vi "Calculate Error.vi"(8 "Rear Right":T1, 9 "Rear Left":T1, 10 "Front Left":T1, 11 "Front Right":T1) -> (0 "Rear Right Angle Error":dbl, 1 "Rear Left Angle Error":dbl, 2 "Rear Right Drive Power":dbl, 3 "Rear Left Drive Power":dbl, 4 "Front Left Angle Error":dbl, 5 "Front Left Drive Power":dbl, 6 "Front Right Angle Error":dbl, 7 "Front Right Drive Power":dbl)   [LabVIEW 2018]
uses:
  Final Motor Data.ctl
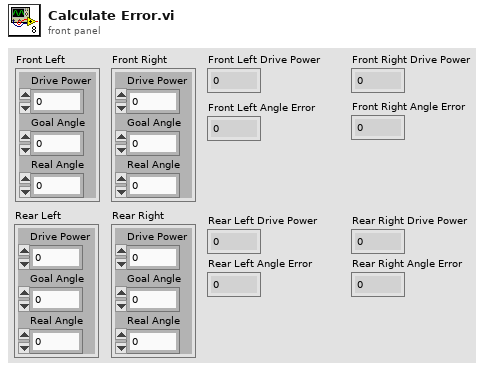
[diagram p1: front panel]
types:
  T1 = typedef "Final Motor Data.ctl" = cluster{"Drive Power":dbl, "Goal Angle":dbl, "Real Angle":dbl}
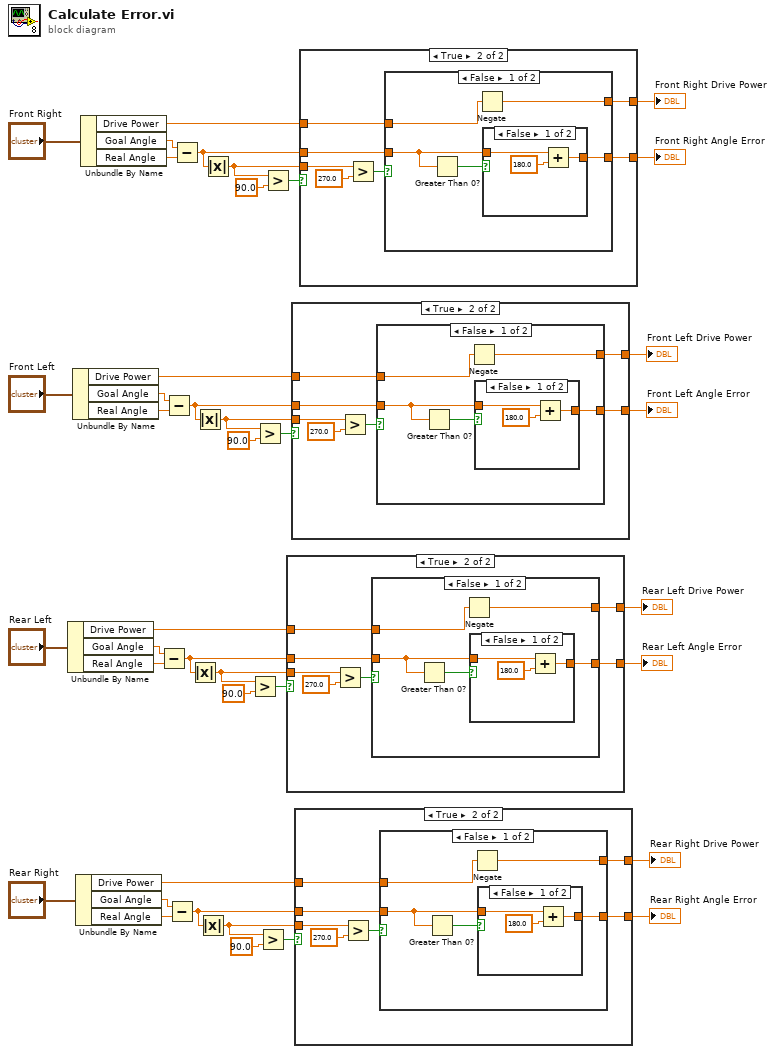
[diagram p0: block diagram]
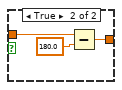
[diagram p3: hidden frame]
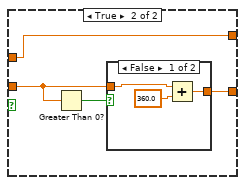
[diagram p4: hidden frame]
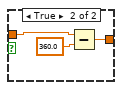
[diagram p5: hidden frame]
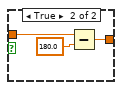
[diagram p7: hidden frame]
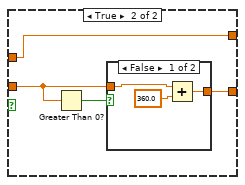
[diagram p8: hidden frame]
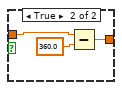
[diagram p9: hidden frame]
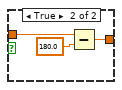
[diagram p11: hidden frame]
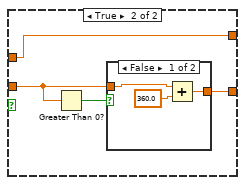
[diagram p12: hidden frame]
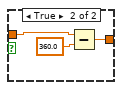
[diagram p13: hidden frame]
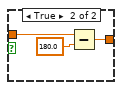
[diagram p15: hidden frame]
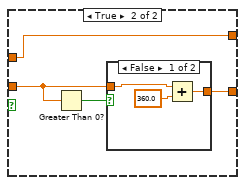
[diagram p16: hidden frame]
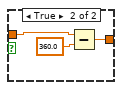
[diagram p17: hidden frame]
diagram:
  n1 = Unbundle By Name("Rear Left") -> ("Drive Power"=w6:dbl, "Goal Angle"=w5:dbl, "Real Angle"=w4:dbl)
  n2 = Unbundle By Name("Front Left") -> ("Drive Power"=w9:dbl, "Goal Angle"=w8:dbl, "Real Angle"=w7:dbl)
  n3 = Unbundle By Name("Rear Right") -> ("Drive Power"=w3:dbl, "Goal Angle"=w2:dbl, "Real Angle"=w1:dbl)
  n4 = Unbundle By Name("Front Right") -> ("Drive Power"=w10:dbl, "Goal Angle"=w12:dbl, "Real Angle"=w11:dbl)
  n5 = Subtract(x=w5, y=w4) -> (x-y=w21:dbl)
  n6 = Subtract(x=w8, y=w7) -> (x-y=w27:dbl)
  n7 = Subtract(x=w2, y=w1) -> (x-y=w15:dbl)
  n8 = Subtract(x=w12, y=w11) -> (x-y=w33:dbl)
  n9 = Absolute Value(x=w21) -> (abs(x)=w22:dbl)
  n10 = Absolute Value(x=w27) -> (abs(x)=w28:dbl)
  n11 = Absolute Value(x=w15) -> (abs(x)=w16:dbl)
  n12 = Absolute Value(x=w33) -> (abs(x)=w34:dbl)
  n13 = Greater?(x=w22, y=90.0) -> (0:w23:bool)
  n14 = Greater?(x=w28, y=90.0) -> (0:w29:bool)
  n15 = Greater?(x=w16, y=90.0) -> (0:w17:bool)
  n16 = Greater?(x=w34, y=90.0) -> (0:w35:bool)
  n17 = case shown="True" w23 {
    tunnel: w22 -> [_ w49]
    tunnel: w6 -> [w42 w46]
    tunnel: [w42 w43] -> w20
    tunnel: [w41 w44] -> w19
    tunnel: w21 -> [w41 w45]
    frame False {
      # "Choice D: NO CHANGE"
    }
    frame True {
      n18 = Greater?(x=w49, y=270.0) -> (0:w47:bool)
      n19 = case shown="False" w47 {
        tunnel: w46 -> [w54 w61]
        tunnel: w45 -> [w51 w63]
        tunnel: [w50 w62] -> w44
        tunnel: [w53 w61] -> w43
        frame False {
          n20 = Greater Than 0?(x=w51) -> (x > 0?=w52:bool)
          n21 = Negate(x=w54) -> (-x=w53:dbl)
          n22 = case shown="False" w52 {
            tunnel: w51 -> [w56 w59]
            tunnel: [w55 w58] -> w50
            frame False {
              n23 = Add(x=w56, y=180.0) -> (x+y=w55:dbl)
            }
            frame True {
              n24 = Subtract(x=w59, y=180.0) -> (x-y=w58:dbl)
            }
          }
        }
        frame True {
          n25 = Greater Than 0?(x=w63) -> (x > 0?=w64:bool)
          n26 = case shown="False" w64 {
            tunnel: w63 -> [w66 w69]
            tunnel: [w65 w68] -> w62
            frame False {
              n27 = Add(x=w66, y=360.0) -> (x+y=w65:dbl)
            }
            frame True {
              n28 = Subtract(x=w69, y=360.0) -> (x-y=w68:dbl)
            }
          }
        }
      }
    }
  }
  "Rear Left Drive Power" <- w20
  "Rear Left Angle Error" <- w19
  n29 = case shown="True" w29 {
    tunnel: w28 -> [_ w79]
    tunnel: w9 -> [w72 w76]
    tunnel: [w72 w73] -> w26
    tunnel: [w71 w74] -> w25
    tunnel: w27 -> [w71 w75]
    frame False {
      # "Choice D: NO CHANGE"
    }
    frame True {
      n30 = Greater?(x=w79, y=270.0) -> (0:w77:bool)
      n31 = case shown="False" w77 {
        tunnel: w76 -> [w84 w91]
        tunnel: w75 -> [w81 w93]
        tunnel: [w80 w92] -> w74
        tunnel: [w83 w91] -> w73
        frame False {
          n32 = Greater Than 0?(x=w81) -> (x > 0?=w82:bool)
          n33 = Negate(x=w84) -> (-x=w83:dbl)
          n34 = case shown="False" w82 {
            tunnel: w81 -> [w86 w89]
            tunnel: [w85 w88] -> w80
            frame False {
              n35 = Add(x=w86, y=180.0) -> (x+y=w85:dbl)
            }
            frame True {
              n36 = Subtract(x=w89, y=180.0) -> (x-y=w88:dbl)
            }
          }
        }
        frame True {
          n37 = Greater Than 0?(x=w93) -> (x > 0?=w94:bool)
          n38 = case shown="False" w94 {
            tunnel: w93 -> [w96 w99]
            tunnel: [w95 w98] -> w92
            frame False {
              n39 = Add(x=w96, y=360.0) -> (x+y=w95:dbl)
            }
            frame True {
              n40 = Subtract(x=w99, y=360.0) -> (x-y=w98:dbl)
            }
          }
        }
      }
    }
  }
  "Front Left Drive Power" <- w26
  "Front Left Angle Error" <- w25
  n41 = case shown="True" w17 {
    tunnel: w16 -> [_ w109]
    tunnel: w3 -> [w102 w106]
    tunnel: [w102 w103] -> w14
    tunnel: [w101 w104] -> w13
    tunnel: w15 -> [w101 w105]
    frame False {
      # "Choice D: NO CHANGE"
    }
    frame True {
      n42 = Greater?(x=w109, y=270.0) -> (0:w107:bool)
      n43 = case shown="False" w107 {
        tunnel: w106 -> [w114 w121]
        tunnel: w105 -> [w111 w123]
        tunnel: [w110 w122] -> w104
        tunnel: [w113 w121] -> w103
        frame False {
          n44 = Greater Than 0?(x=w111) -> (x > 0?=w112:bool)
          n45 = Negate(x=w114) -> (-x=w113:dbl)
          n46 = case shown="False" w112 {
            tunnel: w111 -> [w116 w119]
            tunnel: [w115 w118] -> w110
            frame False {
              n47 = Add(x=w116, y=180.0) -> (x+y=w115:dbl)
            }
            frame True {
              n48 = Subtract(x=w119, y=180.0) -> (x-y=w118:dbl)
            }
          }
        }
        frame True {
          n49 = Greater Than 0?(x=w123) -> (x > 0?=w124:bool)
          n50 = case shown="False" w124 {
            tunnel: w123 -> [w126 w129]
            tunnel: [w125 w128] -> w122
            frame False {
              n51 = Add(x=w126, y=360.0) -> (x+y=w125:dbl)
            }
            frame True {
              n52 = Subtract(x=w129, y=360.0) -> (x-y=w128:dbl)
            }
          }
        }
      }
    }
  }
  "Rear Right Drive Power" <- w14
  "Rear Right Angle Error" <- w13
  n53 = case shown="True" w35 {
    tunnel: w34 -> [_ w139]
    tunnel: w10 -> [w132 w136]
    tunnel: [w132 w133] -> w32
    tunnel: [w131 w134] -> w31
    tunnel: w33 -> [w131 w135]
    frame False {
      # "Choice D: NO CHANGE"
    }
    frame True {
      n54 = Greater?(x=w139, y=270.0) -> (0:w137:bool)
      n55 = case shown="False" w137 {
        tunnel: w136 -> [w144 w151]
        tunnel: w135 -> [w141 w153]
        tunnel: [w140 w152] -> w134
        tunnel: [w143 w151] -> w133
        frame False {
          n56 = Greater Than 0?(x=w141) -> (x > 0?=w142:bool)
          n57 = Negate(x=w144) -> (-x=w143:dbl)
          n58 = case shown="False" w142 {
            tunnel: w141 -> [w146 w149]
            tunnel: [w145 w148] -> w140
            frame False {
              n59 = Add(x=w146, y=180.0) -> (x+y=w145:dbl)
            }
            frame True {
              n60 = Subtract(x=w149, y=180.0) -> (x-y=w148:dbl)
            }
          }
        }
        frame True {
          n61 = Greater Than 0?(x=w153) -> (x > 0?=w154:bool)
          n62 = case shown="False" w154 {
            tunnel: w153 -> [w156 w159]
            tunnel: [w155 w158] -> w152
            frame False {
              n63 = Add(x=w156, y=360.0) -> (x+y=w155:dbl)
            }
            frame True {
              n64 = Subtract(x=w159, y=360.0) -> (x-y=w158:dbl)
            }
          }
        }
      }
    }
  }
  "Front Right Drive Power" <- w32
  "Front Right Angle Error" <- w31
